vi "Virtual shutter close on live imaging stop.vi"(8 "error in (no error)":errorcluster) -> (0 "error out":errorcluster)   [LabVIEW 2020]
uses:
  Typedefs/Read Write Enum.ctl
  Global Variables/General Globals.vi
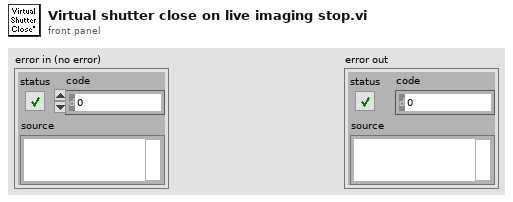
[diagram p1: front panel]
types:
  T1 = typedef "Read Write Enum.ctl" = enum16{"Read", "Write"}
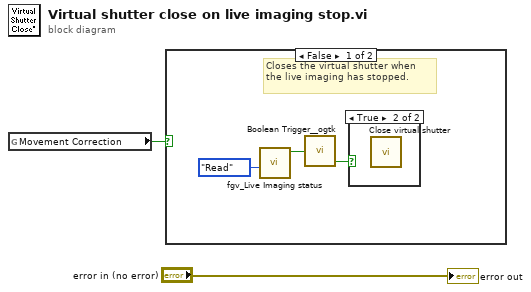
[diagram p0: block diagram]
diagram:
  n1 = global read "General Globals.vi" "Movement Correction"() -> (w1:bool)
  n2 = case shown="False" w1 {
    frame False {
      # "Closes the virtual shutter when the live imaging has stopped."
      n3 = call "fgv_Live Imaging status.vi"("Function"=Read_Write_Enum."Read") -> ("Live Imaging?"=w3:bool)  [unwired: 9 in, 1 out]
      n4 = call <userlib>:"Boolean Trigger__ogtk.vi"("Boolean Input"=w3) -> ("Falling Edge"=w5:bool)  [unwired: 1 in, 1 out]
      n5 = case shown="True" w5 {
        frame False {
        }
        frame True {
          n6 = call "Close virtual shutter.vi"() -> ()  [unwired: 11 in, 1 out]
        }
      }
    }
    frame True {
    }
  }
  "error out" <- "error in (no error)"
